vi "Tester_Simple_uActor_Echo.vi"() -> ()   [LabVIEW 2021]
uses:
  _TestClasses/Test_uActor_Echo/Test_uActor_Echo.lvclass
  Bin/uFramework.lvlibp/uTransport_Event/uTransport_Event.lvclass
  Bin/uFramework.lvlibp/uTransport/uTransport.lvclass
  Bin/uFramework.lvlibp/uMsg/uMsg.lvclass
  Bin/uFramework.lvlibp/uActor/uActor.lvclass
  Bin/uFramework.lvlibp/uTransport_uActor/uTransport_uActor.lvclass
  U:/Projects/uFramework/Bin/uFramework.lvlibp/uActor/uActor.lvclass
  U:/Projects/uFramework/Bin/uFramework.lvlibp/uTransport/uTransport.lvclass
  U:/Projects/uFramework/Testers/_TestClasses/Test_uActor_Echo/Test_uActor_Echo.lvclass
  Bin/uData.lvlibp/uData.lvclass
  U:/Projects/uFramework/Bin/uFramework.lvlibp/uTransport_Event/uTransport_Event.lvclass
  U:/Projects/uFramework/Bin/uFramework.lvlibp/uTransport_uActor/uTransport_uActor.lvclass
panel:
  out "reply":string
  in  "Command":string
  in  "Show FP (F)":bool=TRUE
  out "Is Alive?":bool
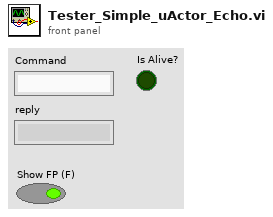
[diagram p1: front panel]
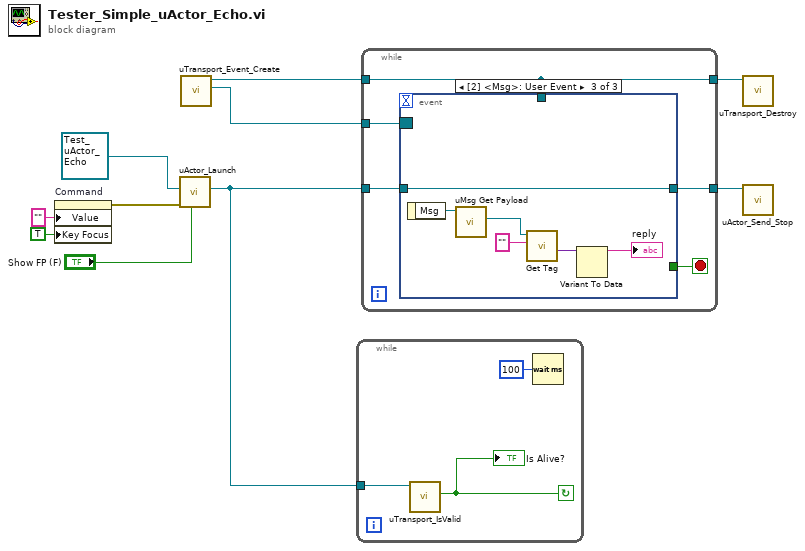
[diagram p0: block diagram]
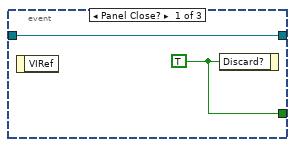
[diagram p2: hidden frame]
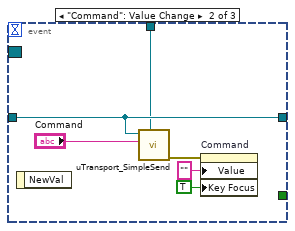
[diagram p3: hidden frame]
diagram:
  n1 = property on="Command" class="Str"("Value"="" ("Command"), "Key Focus"=TRUE) -> (error out=w4:errorcluster)  [unwired: 2 in, 1 out]
  n2 = call "uActor_Launch.vi"("Show FP (F)"="Show FP (F)", "error in (no error)"=w4, "Actor to Launch"=refnum<class "Test_uActor_Echo.lvclass"> refnum ("Class_uActor_Test.lvclass")) -> ("uTransport_uActor"=w7:refnum<class "uTransport_uActor.lvclass">)  [unwired: 6 in, 2 out]
  n3 = call "uTransport_Event_Create.vi"() -> ("Event:uMsg"=w3:refnum<event-registration>, "uTransport_Event out"=w1:refnum<class "uTransport_Event.lvclass">)  [unwired: 9 in, 1 out]
  n4 = while {
    tunnel: w7 -> [w12]
    stop <- w11 continue-if-true
    n5 = call-dynamic "uTransport_IsValid.vi"("uTransport_uActor in"=w12) -> ("IsValid?"=w11:bool)  [unwired: 8 in, 2 out]
    "Is Alive?" <- w11
    n6 = Wait (ms)(milliseconds to wait=u32 100) -> ()  [unwired: 1 out]
  }
  n7 = while {
    tunnel: w7 -> [w17]
    tunnel: [w16] -> w9
    tunnel: w3 -> [w15]
    tunnel: [w14] -> w2
    tunnel: w1 -> [w14]
    stop <- w18 stop-if-true
    n8 = event shown="[2] <Msg>: User Event" {
      selector: w15 -> [_ _ _]
      dyn-events: _ -> [_ _ _]
      timeout: _ -> [_ _ _]
      tunnel: [w20 _ _] -> w18
      tunnel: w17 -> [w19 w26 w32]
      tunnel: [w19 w26 w32] -> w16
      tunnel: w14 -> [_ w21 _]
      event Panel Close? {
        w20 = TRUE ("Discard?")
        n9 = event-data() -> ()  [unwired: 1 in, 1 out]
        n10 = event-data("Discard?"=w20) -> ()  [unwired: 1 in, 1 out]
      }
      event "Command": Value Change {
        n11 = event-data() -> ()  [unwired: 1 in, 1 out]
        n12 = call "uTransport_SimpleSend.vi"("Reply Transport"=w21, "Msg"="Command", "uTransport in"=w26) -> ("error out"=w25:errorcluster)  [unwired: 7 in, 1 out]
        n13 = property on="Command" class="Str"(error in=w25, "Value"="" ("Command"), "Key Focus"=TRUE) -> ()  [unwired: 1 in, 2 out]
      }
      event User Event {
        n14 = event-data() -> ("Msg"=w29:refnum<class "uMsg.lvclass">)  [unwired: 1 in]
        n15 = call "uMsg Get Payload.vi"("uMsg in"=w29) -> ("uData"=w27:refnum<class "uData.lvclass">)  [unwired: 8 in, 2 out]
        n16 = call "Get Tag.vi"("tag (case insensitive)"="", "uData in"=w27) -> ("value"=w31:variant)  [unwired: 6 in, 3 out]
        n17 = Variant To Data(Variant=w31) -> (data=→"reply":string)  [unwired: 2 in, 1 out]
      }
    }
  }
  n18 = call-dynamic "uTransport_Destroy.vi"("uTransport_Event in"=w2) -> ()  [unwired: 10 in, 1 out]
  n19 = call "uActor_Send_Stop.vi"("uActor Transport"=w9) -> ()  [unwired: 10 in, 1 out]
